vi "Sort.vi"(10 "formulas":string[](array[string]), 11 "variables":string[](array[string])) -> (2 "formulas":string[](array[string]), 3 "variables":string[](array[string]))   [LabVIEW 2021, in "d21.lvlib"]
uses:
  d21.lvlib
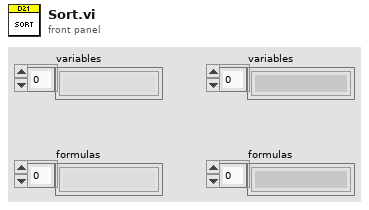
[diagram p1: front panel]
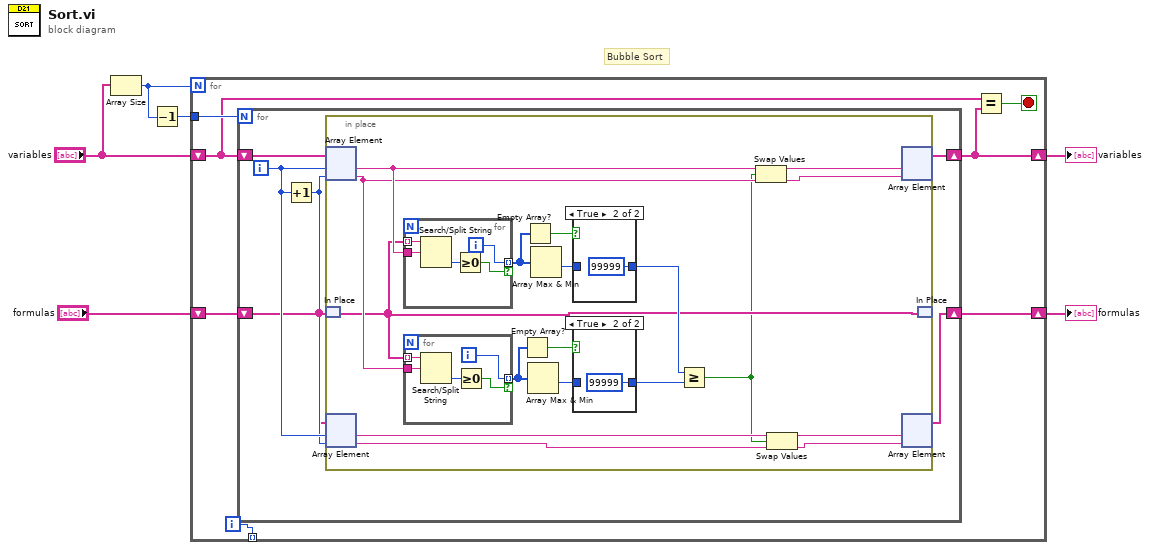
[diagram p0: block diagram]
diagram:
  # "Bubble Sort"
  n1 = Array Size(array="variables") -> (size(s)=w3:i32)
  n2 = Decrement(x=w3) -> (x-1=w1:i32)
  n3 = for {
    N: w3 -> [_]
    tunnel: w1 -> [w12]
    shift-right: [w8] -> w5
    shift-left: "variables" -> [w11]
    shift-right: [w9] -> w6
    shift-left: "formulas" -> [w10]
    tunnel: [w7] -> _ mode=indexing
    i -> [w7]
    stop <- w13 stop-if-true
    n4 = for {
      N: w12 -> [_]
      shift-right: [w18] -> w8
      shift-left: w11 -> [w19]
      shift-right: [w14] -> w9
      shift-left: w10 -> [w15]
      i -> [w17]
      n5 = Increment(x=w17) -> (x+1=w16:i32)
      n6 = in-place {
        n7 = in-place-array #1(w19, w17, w16) -> (w29:string, w28:string)
        n8 = in-place-match #2(w15) -> (w25:string[])
        n9 = in-place-array #3(w15, w17, w16) -> (w24:string, w20:string)
        n10 = for {
          tunnel: [w49] -> w36 mode=indexing if=w50
          tunnel: w29 -> [w48]
          tunnel: w25 -> [w47] mode=indexing
          i -> [w49]
          n11 = Search/Split String(string=w47, search string/char (-)=w48) -> (offset of match=w51:i32)  [unwired: 1 in, 2 out]
          n12 = Greater Or Equal To 0?(x=w51) -> (x >= 0?=w50:bool)
        }
        n13 = for {
          tunnel: [w42] -> w33 mode=indexing if=w43
          tunnel: w28 -> [w41]
          tunnel: w25 -> [w40] mode=indexing
          i -> [w42]
          n14 = Search/Split String(string=w40, search string/char (-)=w41) -> (offset of match=w44:i32)  [unwired: 1 in, 2 out]
          n15 = Greater Or Equal To 0?(x=w44) -> (x >= 0?=w43:bool)
        }
        n16 = Empty Array?(array=w33) -> (empty?=w34:bool)
        n17 = Empty Array?(array=w36) -> (empty?=w37:bool)
        n18 = Array Max & Min(array=w33) -> (min value=w31:i32)  [unwired: 3 out]
        n19 = Array Max & Min(array=w36) -> (min value=w35:i32)  [unwired: 3 out]
        n20 = case shown="True" w37 {
          tunnel: [w45 99999 ("min value")] -> w30
          tunnel: w35 -> [w45 _]
          frame False {
          }
          frame True {
          }
        }
        n21 = case shown="True" w34 {
          tunnel: [w38 99999 ("min value")] -> w32
          tunnel: w31 -> [w38 _]
          frame False {
          }
          frame True {
          }
        }
        n22 = Greater Or Equal?(x=w30, y=w32) -> (x >= y?=w22:bool)
        n23 = Swap Values(12:w29, 13:w22, 14:w28) -> (1:w27:string, 3:w26:string)
        n24 = Swap Values(12:w24, 13:w22, 14:w20) -> (1:w23:string, 3:w21:string)
        n25 = in-place-array #1(w27, w26) -> (w18:string[])  [unwired: 2 out]
        n26 = in-place-array #3(w23, w21) -> (w14:string[])  [unwired: 2 out]
        n27 = in-place-match #2(w25) -> ()  [unwired: 1 out]
      }
    }
    n28 = Equal?(x=w11, y=w8) -> (x = y?=w13:bool)
  }
  "formulas" <- w6
  "variables" <- w5
